vi "Resolve Error.vi"(7 "Formatter (Default)":refnum<class "MultiError Formatter.lvclass">, 9 "MultiErrors in":refnum<class "MultiErrors.lvclass">) -> (1 "MultiErrors out":refnum<class "MultiErrors.lvclass">, 3 "error out":errorcluster)   [LabVIEW 2020, in "VolatusErrorUtilities.lvlib" / "MultiErrors.lvclass"]
uses:
  MultiErrors.lvclass
  MultiError Formatter/MultiError Formatter.lvclass
  MultiErrors.lvclass/MultiErrors.ctl
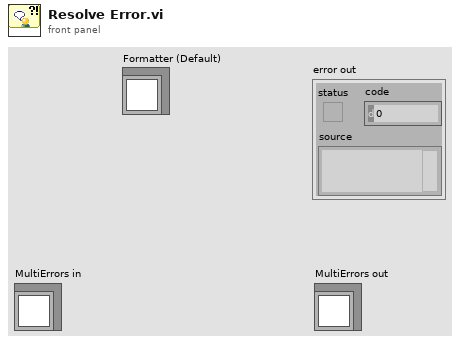
[diagram p1: front panel]
types:
  T1 = typedef "VolatusErrorUtilities.lvlib/MultiError.ctl" = cluster{"Context":string[], "Message":string, "Code":i32, "Call Chain":string[]}
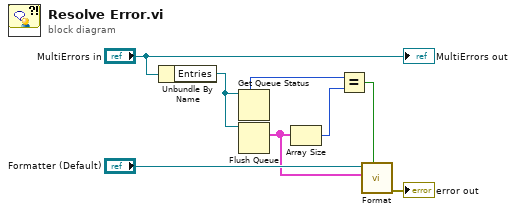
[diagram p0: block diagram]
diagram:
  n1 = Unbundle By Name("MultiErrors in") -> ("Entries"=w7:refnum<queue>)
  n2 = Get Queue Status(queue=w7) -> (max queue size=w6:i32)  [unwired: 2 in, 7 out]
  n3 = Flush Queue(queue=w7) -> (remaining elements=w3:T1[])  [unwired: 1 in, 2 out]
  n4 = Array Size(array=w3) -> (size(s)=w5:i32)
  n5 = Equal?(x=w6, y=w5) -> (x = y?=w2:bool)
  n6 = call "Format.vi"("Max Errors"=w2, "MultiErrors"=w3, "MultiError Formatter in"="Formatter (Default)") -> ("error out"=→"error out":errorcluster)  [unwired: 8 in]
  "MultiErrors out" <- "MultiErrors in"
